vi "OpenStream.vi"(2 "error in (no error)":errorcluster, 3 "StreamID":i32, 4 "IGxDevice":refnum<k24>) -> (0 "error out":errorcluster, 1 "IGxStream":refnum<k24>)   [LabVIEW 2013, in "GxLVlib.lvlib"]
uses:
  GxLVlib.lvlib
  F:/GxILibrary/Labview/trunk/private/dev/src/C#/x64/GxLVLib/dll/GxIAPINET.dll
  private/dev/src/C#/x64/GxLVLib/dll/GxIAPINET.dll
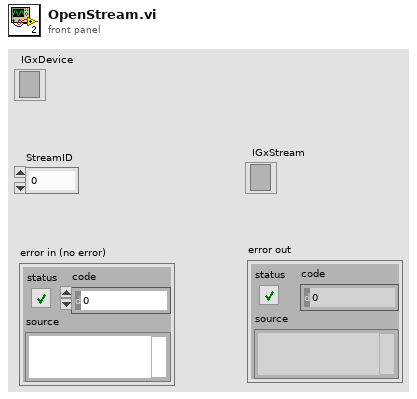
[diagram p1: front panel]
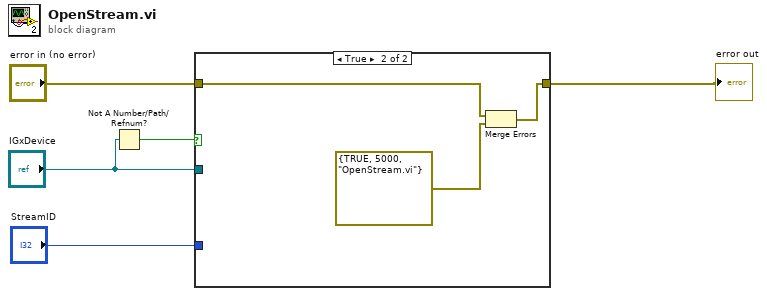
[diagram p0: block diagram]
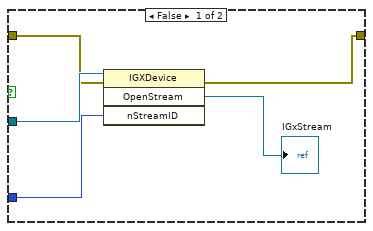
[diagram p2: hidden frame]
diagram:
  n1 = Not A Number/Path/Refnum?(number/path/refnum="IGxDevice") -> (NaN/Path/Refnum?=w5:bool)
  n2 = case shown="True" w5 {
    tunnel: "error in (no error)" -> [w9 w12]
    tunnel: [w7 w11] -> w3
    tunnel: "IGxDevice" -> [w10 _]
    tunnel: "StreamID" -> [w8 _]
    frame False {
      n3 = invoke class="IGXDevice" method="OpenStream"(reference=w10, error in=w9, "nStreamID"=w8) -> (error out=w7:errorcluster, "OpenStream"=→"IGxStream":refnum<k24>)  [unwired: 1 in, 2 out]
    }
    frame True {
      n4 = Merge Errors(w12, errorcluster {TRUE, 5000, "OpenStream.vi"}) -> (w11:errorcluster)
    }
  }
  "error out" <- w3
